vi "UniCODETest.vi"() -> ()   [LabVIEW 2013]
panel:
  in  "Numeric 3":dbl caption="ÿþ8lW[kQÕlABCDE\n\nÛ0ü0à0ðVã–\n\nýVE–‹N¡R"
  in  "Numeric 2":dbl caption="永字八法ABCDE\nホーム困難\n国际事务"
  in  "Numeric":dbl caption="永字八法ABCDE\n???困難\n??事?"
  out "text 3":string
  out "text hex 3":string
  in  "file (use dialog) 3":path
  out "text force UNI 3":string
  out "text hex force UNI 3":string
  out "text 2":string
  out "text hex 2":string
  in  "file (use dialog) 2":path
  out "text force UNI 2":string
  out "text hex force UNI 2":string
  out "text hex force UNI":string
  out "text force UNI":string
  in  "file (use dialog)":path
  out "text hex":string
  out "text":string
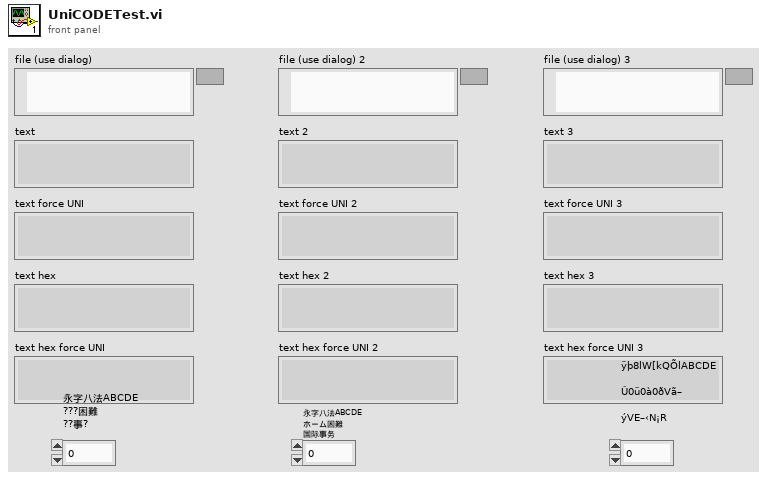
[diagram p1: front panel]
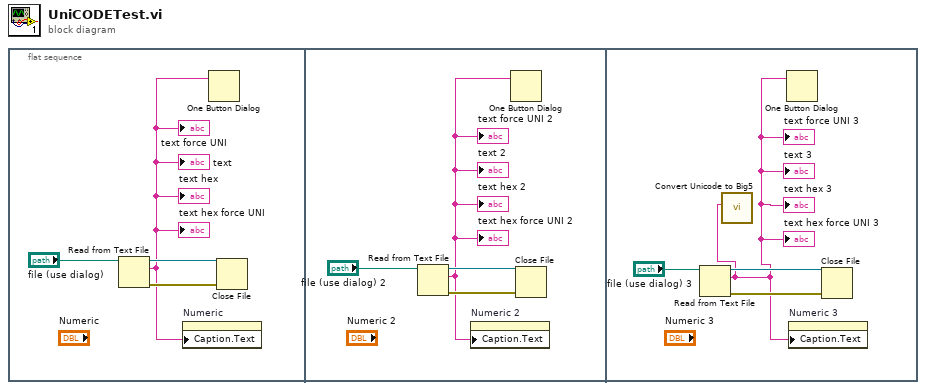
[diagram p0: block diagram]
diagram:
  n1 = flat-sequence {
    frame #0 {
      n2 = Read from Text File(file (use dialog)="file (use dialog)") -> (refnum out=w3:refnum<file>, text=w1:string, error out=w2:errorcluster)  [unwired: 3 in, 1 out]
      "text" <- w1
      "text hex" <- w1
      "text force UNI" <- w1
      "text hex force UNI" <- w1
      n3 = property on="Numeric" class="DigNum (strict)"("Caption.Text"=w1) -> ()  [unwired: 2 in, 2 out]
      n4 = One Button Dialog(message=w1) -> ()  [unwired: 1 in, 1 out]
      n5 = Close File(refnum=w3, error in=w2) -> ()  [unwired: 2 out]
    }
    frame #1 {
      n6 = Read from Text File(file (use dialog)="file (use dialog) 2") -> (refnum out=w8:refnum<file>, text=w5:string, error out=w6:errorcluster)  [unwired: 3 in, 1 out]
      "text 2" <- w5
      "text hex 2" <- w5
      "text force UNI 2" <- w5
      "text hex force UNI 2" <- w5
      n7 = property on="Numeric 2" class="DigNum (strict)"("Caption.Text"=w5) -> ()  [unwired: 2 in, 2 out]
      n8 = One Button Dialog(message=w5) -> ()  [unwired: 1 in, 1 out]
      n9 = Close File(refnum=w8, error in=w6) -> ()  [unwired: 2 out]
    }
    frame #2 {
      n10 = Read from Text File(file (use dialog)="file (use dialog) 3") -> (refnum out=w11:refnum<file>, text=w9:string, error out=w10:errorcluster)  [unwired: 3 in, 1 out]
      "text 3" <- w9
      "text hex 3" <- w9
      "text force UNI 3" <- w9
      "text hex force UNI 3" <- w9
      n11 = call "Convert Unicode to Big5.vi"("UNICODEString"=w9) -> ()  [unwired: 10 in, 1 out]
      n12 = One Button Dialog(message=w9) -> ()  [unwired: 1 in, 1 out]
      n13 = property on="Numeric 3" class="DigNum (strict)"("Caption.Text"=w9) -> ()  [unwired: 2 in, 2 out]
      n14 = Close File(refnum=w11, error in=w10) -> ()  [unwired: 2 out]
    }
  }
